vi "Get Cluster Elements TDs.vi"(8 "错误输入":errorcluster, 10 "Cluster":variant) -> (0 "错误输出":errorcluster, 2 "Type Descriptors":cluster{T1}[](array[cluster]))   [LabVIEW 2012, in "TD Tools.lvlib"]
uses:
  TD Tools.lvlib
  Custom Type/Type Descriptor.ctl
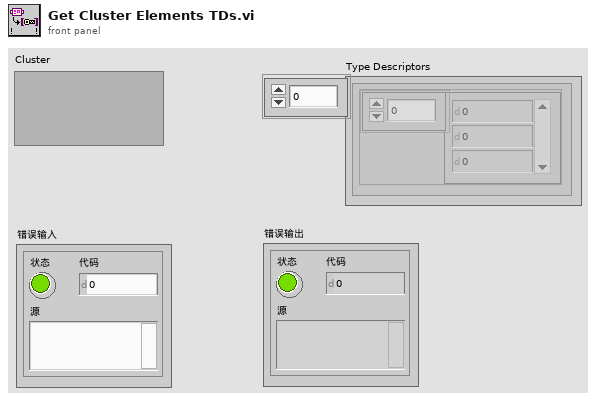
[diagram p1: front panel]
types:
  T1 = typedef "TD Tools.lvlib/Type Descriptor.ctl" = u16[]
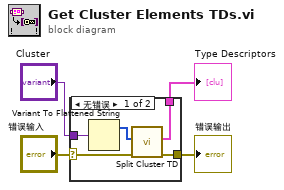
[diagram p0: block diagram]
diagram:
  n1 = case shown="无错误" "错误输入" {
    selector: "错误输入" -> [w8 w10]
    tunnel: [w7 w10] -> w3
    tunnel: "Cluster" -> [w9 _]
    tunnel: [w5 _] -> w1
    frame No Error {
      n2 = Variant To Flattened String(Variant=w9) -> (1:w6:i16[])  [unwired: 1 out]
      n3 = call "Split Cluster TD.vi"("error in (no error)"=w8, "Type Descriptor"=w6) -> ("error out"=w7:errorcluster, "Type Descriptors"=w5:cluster{T1}[])  [unwired: 7 in]
    }
    frame Error {
    }
  }
  "错误输出" <- w3
  "Type Descriptors" <- w1
